vi "Create Fake.vi"(5 "Fake Code Coverage in":refnum<class "Fake Code Coverage.lvclass">, 8 "error in (no error)":errorcluster, 10 "Coverage Percentage":dbl, 11 "All VIs Measured":path[](array[path])) -> (0 "error out":errorcluster, 3 "Fake Code Coverage":refnum<class "Fake Code Coverage.lvclass">)   [LabVIEW 2017, in "Cobertura.Tests.lvlib" / "Fake Code Coverage.lvclass"]
uses:
  Fake Code Coverage.lvclass
  Fake Code Coverage.lvclass/Fake Code Coverage.ctl
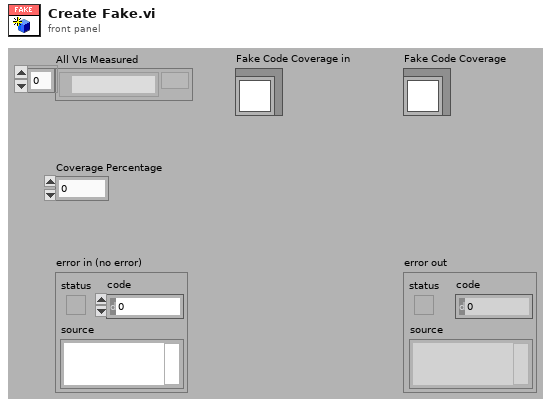
[diagram p1: front panel]
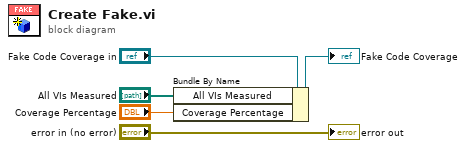
[diagram p0: block diagram]
diagram:
  n1 = Bundle By Name(cluster="Fake Code Coverage in", "All VIs Measured"="All VIs Measured", "Coverage Percentage"="Coverage Percentage") -> (→"Fake Code Coverage":refnum<class "Fake Code Coverage.lvclass">)
  "error out" <- "error in (no error)"
